vi "Set Defaults.vi"(11 "Entity in":refnum<class "Entity.lvclass">) -> (3 "Entity out":refnum<class "Entity.lvclass">)   [LabVIEW 2022 SP3, in "Conditum.lvlib" / "Entity.lvclass"]
uses:
  Entity.lvclass
  Entity.lvclass/Entity.ctl
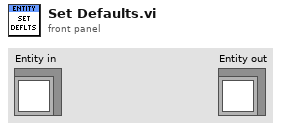
[diagram p1: front panel]
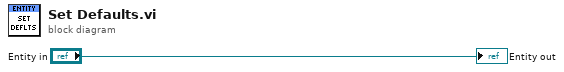
[diagram p0: block diagram]
diagram:
  "Entity out" <- "Entity in"
